vi "ControllaIndice.vi"(10 "Contenuto file 2":string[][](array[string]), 11 "Indice Sensore":i32=2) -> (1 "Sensore Selez.":string, 2 "OK":bool, 3 "Indice Sensore 2":i32)   [LabVIEW 2019]
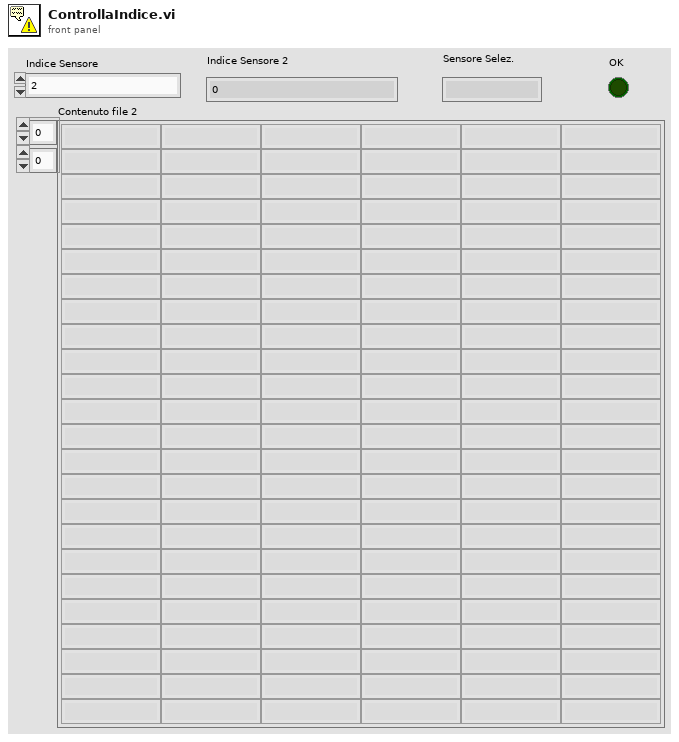
[diagram p1: front panel]
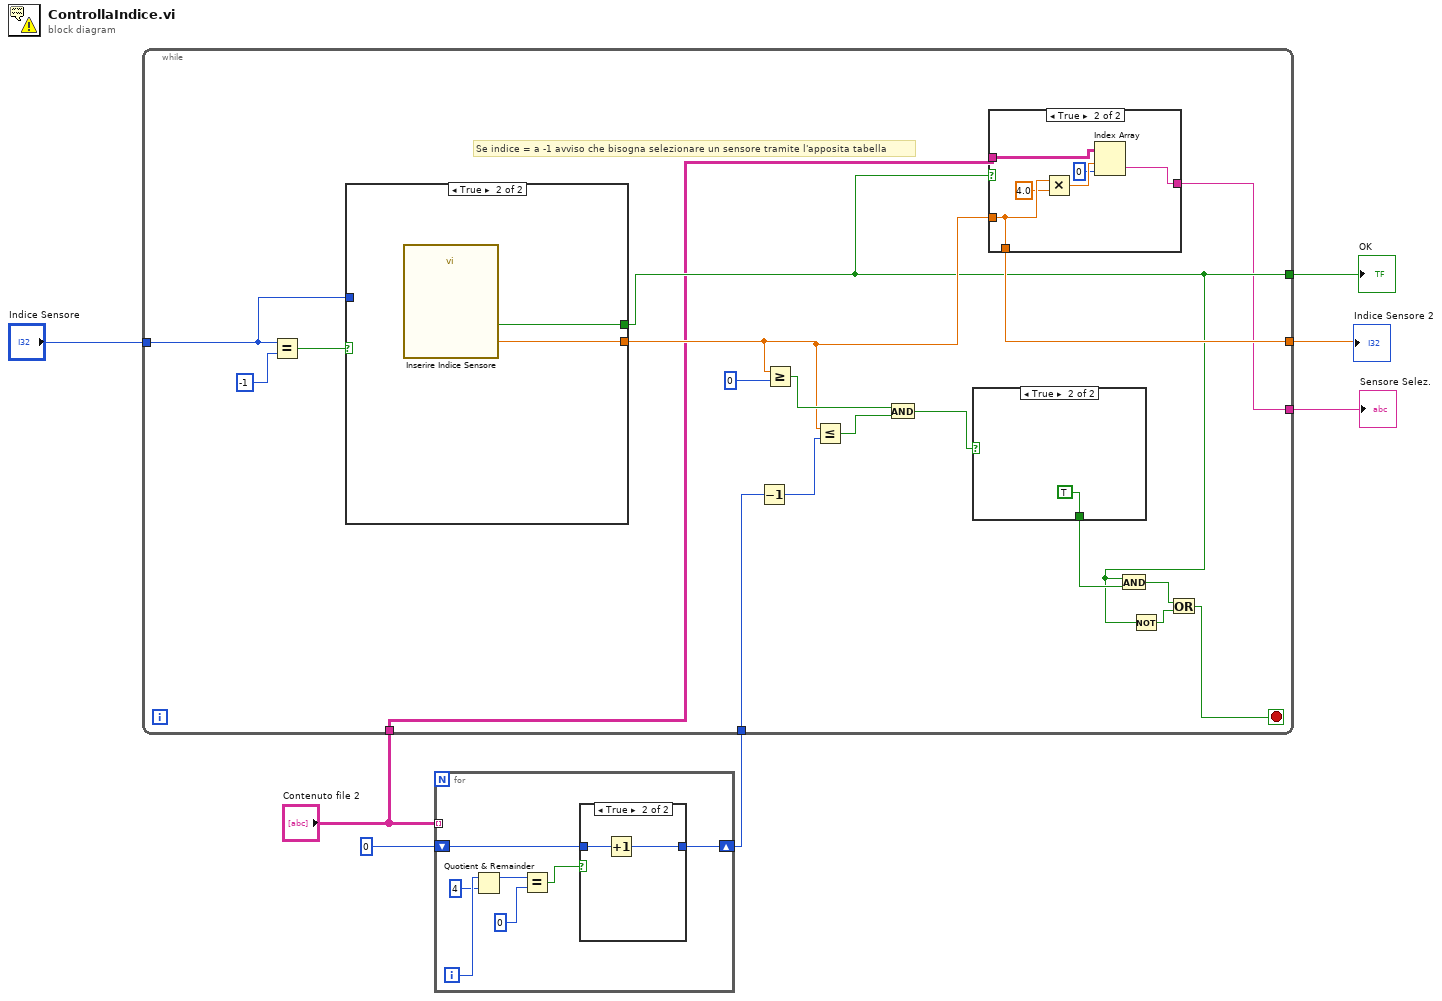
[diagram p0: block diagram]
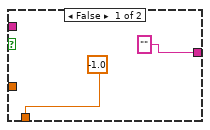
[diagram p3: hidden frame]
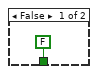
[diagram p4: hidden frame]
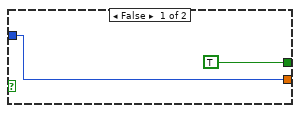
[diagram p5: hidden frame]
diagram:
  n1 = for {
    tunnel: "Contenuto file 2" -> [_] mode=indexing
    shift-right: [w8] -> w5
    shift-left: 0 ("y") -> [w9]
    i -> [w14]
    n2 = Quotient & Remainder(x=w14, y=4) -> (x-y*floor(x/y)=w12:i32)  [unwired: 1 out]
    n3 = Equal?(x=w12, y=0) -> (x = y?=w10:bool)
    n4 = case shown="True" w10 {
      tunnel: w9 -> [w15 w17]
      tunnel: [w15 w16] -> w8
      frame False {
      }
      frame True {
        n5 = Increment(x=w17) -> (x+1=w16:i32)
      }
    }
  }
  n6 = while {
    tunnel: "Indice Sensore" -> [w33]
    tunnel: w5 -> [w32]
    tunnel: [w21] -> w4
    tunnel: [w25] -> w3
    tunnel: "Contenuto file 2" -> [w18]
    tunnel: [w19] -> w1
    stop <- w20 stop-if-true
    # "Se indice = a -1 avviso che bisogna selezionare un sensore tramite l'apposita tabella"
    n7 = Equal?(x=w33, y=-1) -> (x = y?=w34:bool)
    n8 = case shown="True" w34 {
      tunnel: w33 -> [w46 _]
      tunnel: [TRUE ("OK") w49] -> w21
      tunnel: [w46 w48] -> w26
      frame False {
      }
      frame True {
        n9 = call "Inserire Indice Sensore"() -> ("Indice Sensore"=w48:dbl, "OK"=w49:bool)  [unwired: 17 in, 1 out]
      }
    }
    n10 = Decrement(x=w32) -> (x-1=w28:i32)
    n11 = Greater Or Equal?(x=w26, y=0) -> (x >= y?=w30:bool)
    n12 = Less Or Equal?(x=w26, y=w28) -> (x <= y?=w29:bool)
    n13 = And(x=w30, y=w29) -> (x .and. y?=w27:bool)
    n14 = case shown="True" w27 {
      tunnel: [FALSE TRUE] -> w24
      frame False {
      }
      frame True {
      }
    }
    n15 = case shown="True" w21 {
      tunnel: w26 -> [_ w43]
      tunnel: [-1.0 ("Indice Sensore") w43] -> w25
      tunnel: ["" w38] -> w19
      tunnel: w18 -> [_ w41]
      frame False {
      }
      frame True {
        n16 = Multiply(x=w43, y=4.0) -> (x*y=w40:dbl)
        n17 = Index Array(array=w41, index (row)=w40, index (col)=0 ("disabled index (col)")) -> (element=w38:string)
      }
    }
    n18 = And(x=w21, y=w24) -> (x .and. y?=w23:bool)
    n19 = Not(x=w21) -> (.not. x?=w22:bool)
    n20 = Or(x=w23, y=w22) -> (x .or. y?=w20:bool)
  }
  "OK" <- w4
  "Indice Sensore 2" <- w3
  "Sensore Selez." <- w1
